vi "OFBS_read_ClassifierType.vi"(8 "error in (no error)":errorcluster, 11 "OptFreqBandsSearch in":refnum<class "OptFreqBandsSearch.lvclass">) -> (0 "error out":errorcluster, 1 "Classifier Metaparameter":dbl, 2 "ClassifierType":T1, 3 "OptFreqBandsSearch out":refnum<class "OptFreqBandsSearch.lvclass">)   [LabVIEW 2016, in "Optimal Frequency Bands Search.lvlib" / "OptFreqBandsSearch.lvclass"]
uses:
  OptFreqBandsSearch.lvclass
  OFBS_ClassifierTypes.ctl
  OptFreqBandsSearch.lvclass/OptFreqBandsSearch.ctl
  Optimal Frequency Bands Search.lvlib
panel:
  # "This VI is a part of BCI Design library, http://www.ru-bci.org \nCopyright © 2020, Sotnikov Peter, All rights reserved. License: GNU GPLv3"
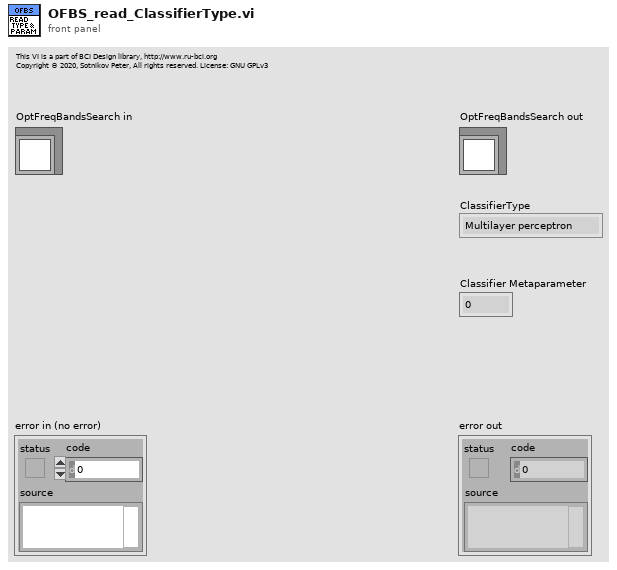
[diagram p1: front panel]
types:
  T1 = typedef "Optimal Frequency Bands Search.lvlib/OFBS_ClassifierTypes.ctl" = enum16{"Multilayer perceptron", "k NN Classifier", "SVM Committee", "Mahalanobis distance", "SVM Classifier"}
  T2 = typedef "Classifier.lvlib/CU_ClassifierTypes.ctl" = enum16{"Multilayer perceptron", "k NN Classifier", "SVM Committee", "Mahalanobis distance", "SVM Classifier"}
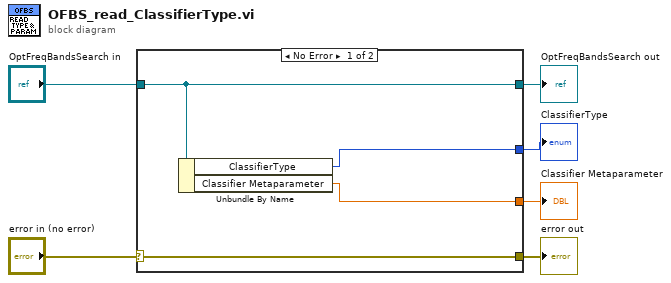
[diagram p0: block diagram]
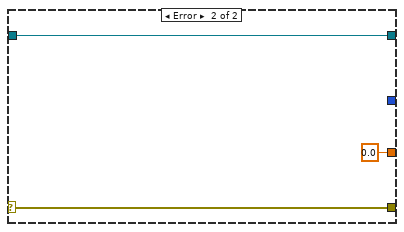
[diagram p2: hidden frame]
diagram:
  n1 = case shown="No Error" "error in (no error)" {
    selector: "error in (no error)" -> [w10 w12]
    tunnel: [w10 w12] -> w5
    tunnel: [w9 w13] -> w3
    tunnel: "OptFreqBandsSearch in" -> [w9 w13]
    tunnel: [w8 _] -> w2
    tunnel: [w7 0.0 ("Classifier Metaparameter")] -> w1
    frame No Error {
      n2 = Unbundle By Name(w9) -> ("ClassifierType"=w8:T2, "Classifier Metaparameter"=w7:dbl)
    }
    frame Error {
    }
  }
  "error out" <- w5
  "OptFreqBandsSearch out" <- w3
  "ClassifierType" <- w2
  "Classifier Metaparameter" <- w1
